vi "AB_Long_Path_Error.vi"(8 "error in (no error)":errorcluster, 9 "Maximum Allowable Path Length (252)":i32=252, 10 "Path":path, 11 "error string in":string) -> (0 "error out":errorcluster, 3 "error string out":string)   [LabVIEW 2020]
uses:
  <resource>/Framework/Providers/Common/provcom_StringGlobals.vi
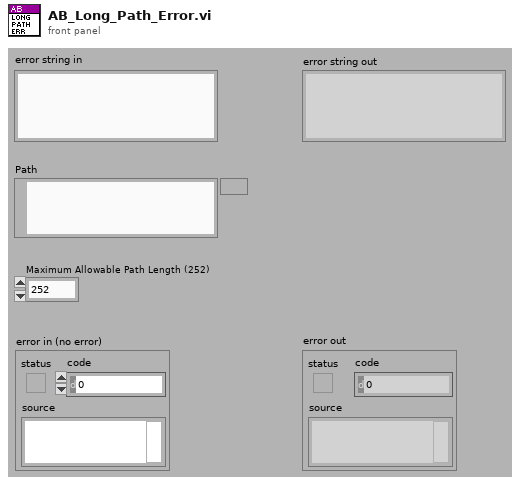
[diagram p1: front panel]
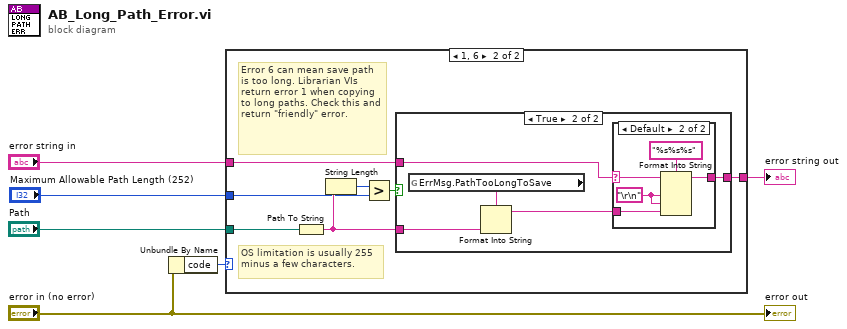
[diagram p0: block diagram]
diagram:
  n1 = Unbundle By Name("error in (no error)") -> ("code"=w3:i32)
  n2 = case shown="1, 6" w3 {
    tunnel: "error string in" -> [w7 w14]
    tunnel: [w7 w13] -> w6
    tunnel: "Path" -> [_ w9]
    tunnel: "Maximum Allowable Path Length (252)" -> [_ w8]
    frame Default {
    }
    frame 1, 6 {
      # "OS limitation is usually 255 minus a few characters."
      # "Error 6 can mean save path is too long. Librarian VIs return error 1 when copying to long paths. Check this and return \"friendly\" error."
      n3 = Path To String(path=w9) -> (string=w11:string)
      n4 = String Length(string=w11) -> (length=w12:i32)
      n5 = Greater?(x=w12, y=w8) -> (0:w10:bool)
      n6 = case shown="True" w10 {
        tunnel: w14 -> [w15 w16]
        tunnel: [w15 w20] -> w13
        tunnel: w11 -> [_ w17]
        frame False {
        }
        frame True {
          n7 = global read "provcom_StringGlobals.vi" "ErrMsg.PathTooLongToSave"() -> (w19:string)
          n8 = Format Into String(format string=w19, w17) -> (resulting string=w18:string)  [unwired: 2 in, 1 out]
          n9 = case shown="Default" w16 {
            selector: w16 -> [_ w23]
            tunnel: [w21 w25] -> w20
            tunnel: w18 -> [w21 w24]
            frame "" {
            }
            frame Default {
              w22 = "\r\n"
              n10 = Format Into String(format string="%s%s%s", initial string=w23, w22, w22, w24) -> (resulting string=w25:string)  [unwired: 1 in, 1 out]
            }
          }
        }
      }
    }
  }
  "error string out" <- w6
  "error out" <- "error in (no error)"
